vi "Start Triggers Sync PPS Trig Core.vi"(0 "sync.resources":T2, 1 "rx 0.stream enable":bool, 2 "rx 1.stream enable":bool, 3 "tx 0.stream enable":bool, 4 "tx 1.stream enable":bool, 6 "rx.trigger select":T1=enum."Immediate", 7 "tx.trigger select":T1=enum."Immediate", 8 "rx.software trigger":bool, 9 "tx.software trigger":bool, 10 "rx.trigger enable":bool, 11 "tx.trigger enable":bool, 12 "rx.trigger sync enable":bool, 13 "tx.trigger sync enable":bool) -> (14 "rx.start trigger":bool, 15 "tx.start trigger":bool)   [LabVIEW 2023]
uses:
  <instrlib>/niUSRPRIO/Synchronization/v1/FPGA/niUsrpRio Synchronization v1 FPGA.lvlib
  <instrlib>/niUSRPRIO/Synchronization/v1/FPGA/Private/Synchronize over PPS Trig.vi
  <instrlib>/niUSRPRIO/Synchronization/v1/FPGA/Private/Resources.ctl
  <instrlib>/niVST/Reference FPGA/FPGA/USRPRIO Sample VIs/Host/SubVIs/Start Trigger.ctl
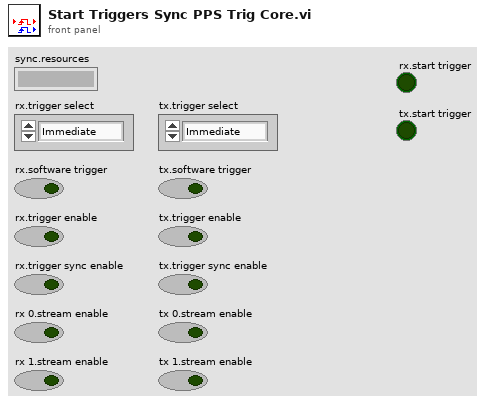
[diagram p1: front panel]
types:
  T1 = typedef "Start Trigger.ctl" = enum8{"Software", "Digital Edge", "Rx Start Trigger", "Tx Start Trigger", "Immediate", "Future Time Event"}
  T2 = typedef "niUsrpRio Synchronization v1 FPGA.lvlib/Resources.ctl" = cluster{"master":refnum<k21>, "meas.enable":refnum<k21>, "meas.ready":refnum<k21>, "meas.reset":refnum<k21>, "meas.arm":refnum<k21>, "meas.valid":refnum<k21>, "meas.value":refnum<k21>, "meas.oversample factor":refnum<k21>, "cptr":refnum<k21>, "cptr.adjust":refnum<k21>, "cptr.period":refnum<k21>}
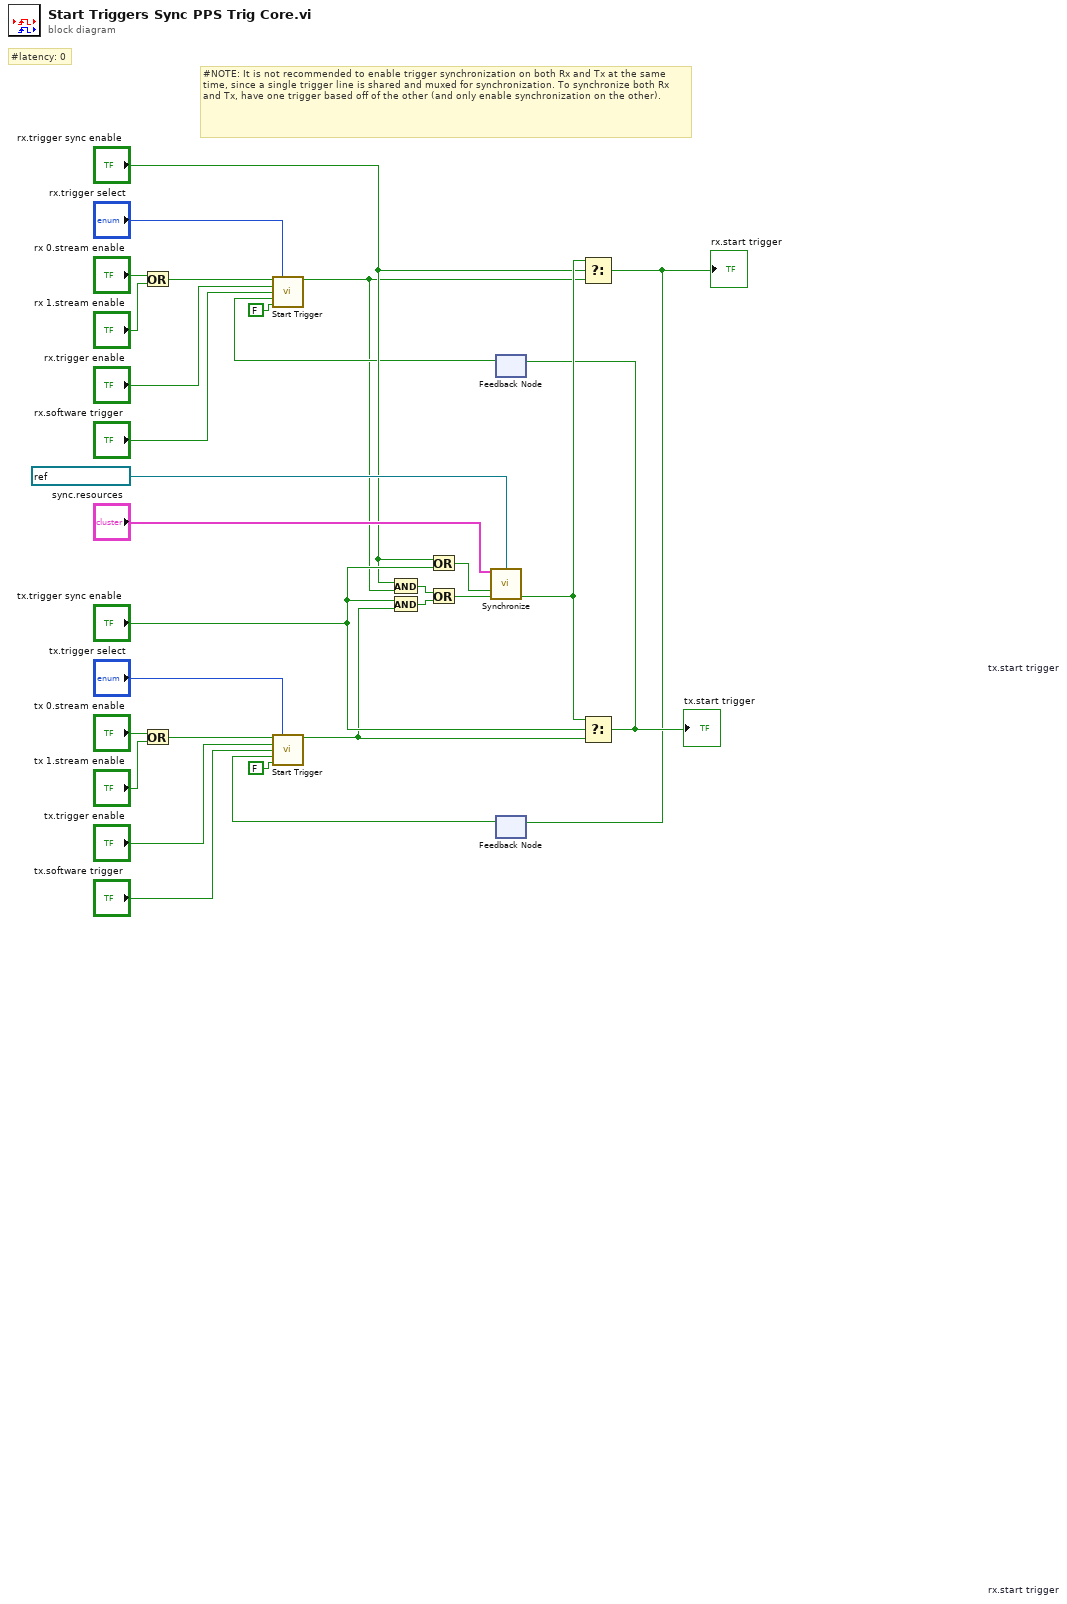
[diagram p0: block diagram]
diagram:
  # "#latency: 0"
  # "#NOTE: It is not recommended to enable trigger synchronization on both Rx and Tx at the same time, since a single trigger line is shared and muxed for synchronization. To synchronize both Rx and Tx, have one trigger based off of the other (and only enable synchronization on the other)."
  n1 = Or(x="rx 0.stream enable", y="rx 1.stream enable") -> (x .or. y?=w5:bool)
  n2 = Or(x="tx 0.stream enable", y="tx 1.stream enable") -> (x .or. y?=w29:bool)
  n3 = Or(x="rx.trigger sync enable", y="tx.trigger sync enable") -> (x .or. y?=w24:bool)
  n4 = feedback #1 "tx.start trigger"() -> (w11:bool)  [unwired: 1 in]
  n5 = call <instrlib>:"Start Trigger.vi"("stream enable"=w5, "trigger select"="rx.trigger select", "trigger enable"="rx.trigger enable", "software trigger"="rx.software trigger", "other start trigger"=w11, "event occurred"=FALSE) -> ("start trigger"=w10:bool)  [unwired: 9 in]
  n6 = And(x="rx.trigger sync enable", y=w10) -> (x .and. y?=w16:bool)
  n7 = feedback #2 "rx.start trigger"() -> (w7:bool)  [unwired: 1 in]
  n8 = call <instrlib>:"Start Trigger.vi"("stream enable"=w29, "trigger select"="tx.trigger select", "trigger enable"="tx.trigger enable", "software trigger"="tx.software trigger", "other start trigger"=w7, "event occurred"=FALSE) -> ("start trigger"=w9:bool)  [unwired: 9 in]
  n9 = And(x="tx.trigger sync enable", y=w9) -> (x .and. y?=w18:bool)
  n10 = Or(x=w16, y=w18) -> (x .or. y?=w22:bool)
  n11 = call-poly <instrlib>:"Synchronize.vi"("sync.resources"="sync.resources", "clock x2"=refnum<k21> "Data Clock x2", "enable"=w24, "edge"=w22) -> ("synchronized edge"=w23:bool)  [unwired: 9 in, 2 out]
  n12 = Select(t=w23, s="rx.trigger sync enable", f=w10) -> (s? t:f=w1:bool)
  "rx.start trigger" <- w1
  n13 = feedback-in #2(w1) -> ()
  n14 = Select(t=w23, s="tx.trigger sync enable", f=w9) -> (s? t:f=w2:bool)
  "tx.start trigger" <- w2
  n15 = feedback-in #1(w2) -> ()
